vi "Create Temp Sensor Object.vi"(8 "error in (no error)":errorcluster, 11 "LCM Single-Up MTS Test in":refnum<class "LCM Single-Up MTS Test.lvclass">) -> (0 "error out":errorcluster, 3 "ThorLabs TSP01 out":refnum<class "ThorLabs TSP01.lvclass">)   [LabVIEW 2015, in "LCM Single-Up MTS Test.lvclass"]
uses:
  LCM Single-Up MTS Test.lvclass
  Classes/Instruments/Temperature Device/ThorLabs TSP01/Class/ThorLabs TSP01.lvclass
  CBTF Applications/SmartCast Testing/Main/LCM Single-Up/Application/Application/Class/typedefs/Instrument Selector -- Enum.ctl
  Test Class/Test Class.lvclass
  CBTF Applications/SmartCast Testing/Main/LCM Single-Up/Application/Application/Class/LCM Single-Up.lvclass
  Classes/Application/Class/Application.lvclass
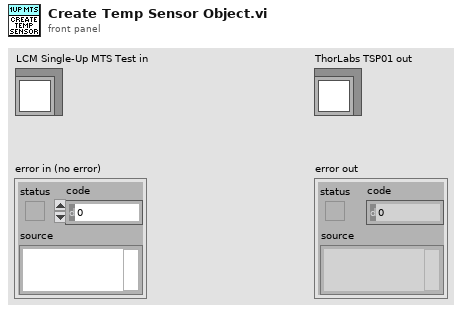
[diagram p1: front panel]
types:
  T1 = typedef "LCM Single-Up.lvlib/LCM Single-Up.lvclass/Instrument Selector -- Enum.ctl" = enum16{"Relay", "MIO Device", "I2C Device", "Thermocouple"}
  T2 = typedef "Application.lvlib/App Properties.lvclass/Class Properties -- Cluster.ctl" = cluster{"UUT Info":T3[], "Test Information":refnum<vi>, "Test Complete Event":refnum<user-event>, "Shop Floor System":refnum<class "Shop Floor System.lvclass">, "Gold Board":refnum<class "Golden Board.lvclass">, "Test Recipe":refnum<class "Test Recipe.lvclass">, "Instruments":refnum<class "Base Class.lvclass">[], "Mode":T4, "Test Results":cluster{"Pass":bool[], "Fail Codes":string[]}, "Station Config":refnum<class "Station Config.lvclass">}
  T3 = typedef "Application.lvlib/App Properties.lvclass/UUT Reference -- Cluster.ctl" = cluster{"Serial Number Reference":refnum<vi>, "Status Message Reference":refnum<vi>}
  T4 = typedef "Application.lvlib/Application.lvclass/Op Mode -- Enum.ctl" = u16
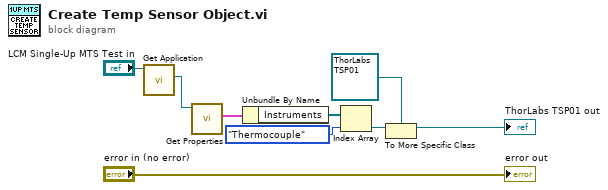
[diagram p0: block diagram]
diagram:
  n1 = call "Get Application.vi"("Test Class in"="LCM Single-Up MTS Test in") -> ("Application.lvlib:Application.lvclass"=w1:refnum<class "Application.lvclass">)  [unwired: 9 in, 1 out]
  n2 = call "Get Properties.vi"("Acrobat Template in"=w1) -> ("Class Properties"=w6:T2)  [unwired: 8 in, 2 out]
  n3 = Unbundle By Name(w6) -> ("Instruments"=w8:refnum<class "Base Class.lvclass">[])
  n4 = Index Array(array=w8, index=Instrument_Selector_--_Enum."Thermocouple" ("Instrument")) -> (element=w7:refnum<class "Base Class.lvclass">)
  n5 = To More Specific Class(target class=refnum<class "ThorLabs TSP01.lvclass"> refnum ("ThorLabs TSP01 out"), reference=w7) -> (specific class reference=→"ThorLabs TSP01 out":refnum<class "ThorLabs TSP01.lvclass">)  [unwired: 1 in, 1 out]
  "error out" <- "error in (no error)"
